vi "catch_calc.vi"(11 "Catch Inputs":T3) -> (3 "Catch Outputs":T1)   [LabVIEW 2013]
uses:
  catch_inputs.ctl
  catch_outputs.ctl
  <vilib>/Rock Robotics/WPI/Solenoid/WPI_SolenoidValue.ctl
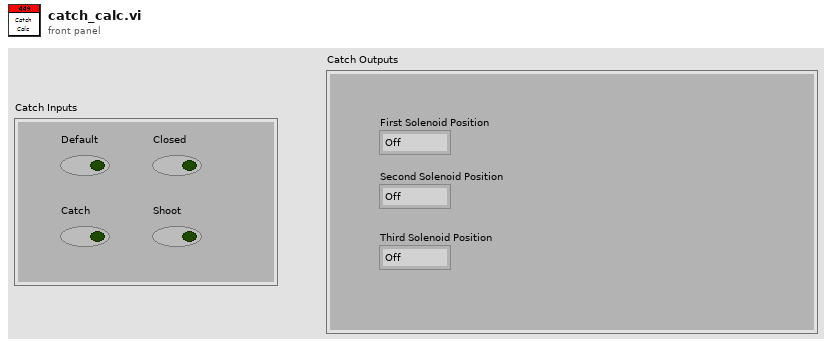
[diagram p1: front panel]
types:
  T1 = typedef "catch_outputs.ctl" = cluster{"First Solenoid Position":T2, "Second Solenoid Position":T2, "Third Solenoid Position":T2}
  T2 = typedef "WPI_SolenoidValue.ctl" = enum16{"Off", "On", "Forward", "Reverse"}
  T3 = typedef "catch_inputs.ctl" = cluster{"Default":bool, "Closed":bool, "Catch":bool, "Shoot":bool}
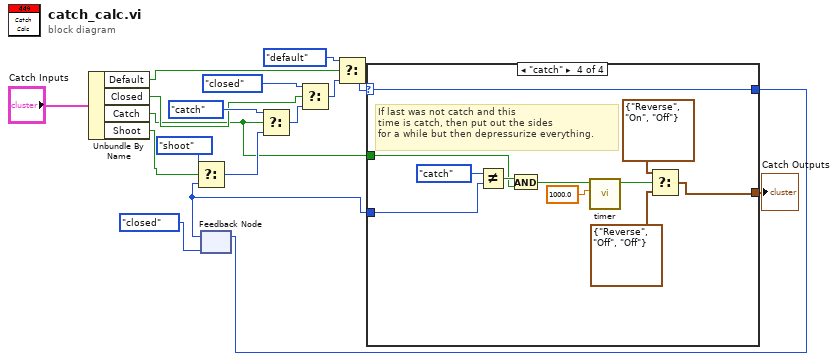
[diagram p0: block diagram]
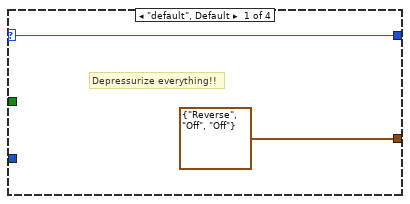
[diagram p2: hidden frame]
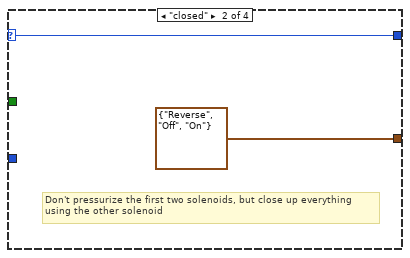
[diagram p3: hidden frame]
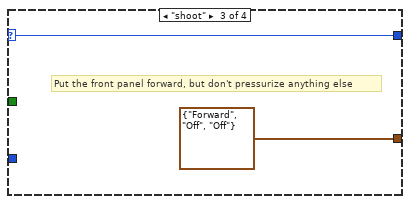
[diagram p4: hidden frame]
diagram:
  n1 = Unbundle By Name("Catch Inputs") -> ("Default"=w8:bool, "Closed"=w11:bool, "Catch"=w1:bool, "Shoot"=w2:bool)
  n2 = feedback #1(enum16{"default", "closed", "shoot", "catch"}."closed") -> (w3:enum16{"default", "closed", "shoot", "catch"})
  n3 = Select(t=enum16{"default", "closed", "shoot", "catch"}."shoot", s=w2, f=w3) -> (s? t:f=w14:enum16{"default", "closed", "shoot", "catch"})
  n4 = Select(t=enum16{"default", "closed", "shoot", "catch"}."catch", s=w1, f=w14) -> (s? t:f=w12:enum16{"default", "closed", "shoot", "catch"})
  n5 = Select(t=enum16{"default", "closed", "shoot", "catch"}."closed", s=w11, f=w12) -> (s? t:f=w9:enum16{"default", "closed", "shoot", "catch"})
  n6 = Select(t=enum16{"default", "closed", "shoot", "catch"}."default", s=w8, f=w9) -> (s? t:f=w6:enum16{"default", "closed", "shoot", "catch"})
  n7 = case shown="\"catch\"" w6 {
    selector: w6 -> [w18 w21 w23 w34]
    tunnel: [w18 w21 w23 w34] -> w5
    tunnel: [T1 {"First Solenoid Position"=enum."Reverse", "Second Solenoid Position"=enum."Off", "Third Solenoid Position"=enum."Off"} ("Catch Outputs") T1 {"First Solenoid Position"=enum."Reverse", "Second Solenoid Position"=enum."Off", "Third Solenoid Position"=enum."On"} ("Catch Outputs") T1 {"First Solenoid Position"=enum."Forward", "Second Solenoid Position"=enum."Off", "Third Solenoid Position"=enum."Off"} ("Catch Outputs") w30] -> w4
    tunnel: w3 -> [_ _ _ w27]
    tunnel: w1 -> [_ _ _ w24]
    frame "default", Default {
      # "Depressurize everything!!"
    }
    frame "closed" {
      # "Don't pressurize the first two solenoids, but close up everything\nusing the other solenoid"
    }
    frame "shoot" {
      # "Put the front panel forward, but don't pressurize anything else"
    }
    frame "catch" {
      # "If last was not catch and this\ntime is catch, then put out the sides\nfor a while but then depressurize everything."
      n8 = Not Equal?(x=enum16{"default", "closed", "shoot", "catch"}."catch", y=w27) -> (x != y?=w26:bool)
      n9 = And(x=w26, y=w24) -> (x .and. y?=w25:bool)
      n10 = call "timer.vi"("Time"=1000.0, "Set"=w25) -> ("Out"=w32:bool)  [unwired: 9 in]
      n11 = Select(t=T1 {"First Solenoid Position"=enum."Reverse", "Second Solenoid Position"=enum."On", "Third Solenoid Position"=enum."Off"} ("Catch Outputs"), s=w32, f=T1 {"First Solenoid Position"=enum."Reverse", "Second Solenoid Position"=enum."Off", "Third Solenoid Position"=enum."Off"} ("Catch Outputs")) -> (s? t:f=w30:T1)
    }
  }
  "Catch Outputs" <- w4
  n12 = feedback-in #1(w5) -> ()
